vi "SPM Pump v0.7.vi"(0 "Termination char\n(0xA = '\\n' = LF)\n(0xD = '\\r' = CR)":u8=13 format="%.0x", 1 "Enable Termination\nChar (T)":bool=TRUE, 2 "Timeout (ms)":u32=10000, 3 "Serial Settings:Serial End Mode for Reads":u16(ring)=2 items=["None", "LastBit", "TermChar"], 4 "byte count":u32=64, 5 "Delay before read (ms)":u32=1000, 6 "Time <input>":dbl, 7 "error in (no error)":errorcluster, 8 "Serial port input":string="/1ZR", 9 "VISA resource name":refnum<visa-resource-name>="COM6", 10 "parity":u16(ring) items=["None", "Odd", "Even", "Mark", "Space"], 11 "baud rate":u32=9600, 12 "stop bits":u16(ring)=10 items=["1.0"=10, "1.5"=15, "2.0"=20], 13 "data bits":u16=8 min=5 max=8 step=1, 14 "flow control":u16(ring) items=["None"=0, "XON/XOFF"=1, "RTS/CTS"=2, "DTR/DSR"=4], 15 "Time units <input>":string, 19 "Hard stop pump":bool, 20 "Halt pump":bool) -> (16 "Input command":string, 17 "Serial port data":string[](array[string]), 18 "Pump status":string, 23 "Valve position":i32, 24 "Absolute plunger position":i32, 25 "Actual plunger position":i32, 26 "Serial port":string, 27 "error out":errorcluster)   [LabVIEW 2019]
doc: "The Basic Serial Read and Write example performs a Serial Port Read, a Serial Port Write, or a combination of these actions. The user selects the actions (read or write) on the front panel. If both are selected, the VI will write the data first, read data, and then close the VISA session that is opened to the port. This VI will wait until the specified number of bytes is received at the port. Only the number of bytes specified will be read.\n\nINSTRUCTIONS:\n1) Select the serial resource and configuration parameters (baud rate, data bits, parity, stop bits, flow control).\n2) Select the operations to be performed. \n3) Connect the serial port to your device. If no device is available, perform a loopback test by doing one of the following. Short pins 2 and 3 on a RS-232 cable or short pin 4 to pin 8 and pin 5 to pin 9 on a RS-485/422 cable. \n4) Run the VI to see the data read. (The \"read string\" will match the \"string to write\" if a loopback test was performed.)\n\nNote: The parameters set for the serial port must match the parameters of the connected instrument or device. In this example, the bytes to read parameter specifies the number of bytes that the serial port reads. If there were more bytes at the port than the number specified in bytes to read, those bytes would not be read. Also, if you specify to read more bytes than the number of bytes actually read, you might receive a timeout error message.\n\nOn the block diagram, the Configure Serial Port VI sets the configuration parameters. The front panel displays the controls used to configure the basic parameters, such as baud rate, data bits, and parity. Constants configure the other parameters the user probably does not need set. After the VISA Configure Serial Port VI opens the VISA session and configures the port, the VI passes the VISA resource name to other VIs that perform operations on that VISA resource. The VISA Write function sends a command to the serial device and the VISA Read function returns data based on the command. The VISA Close function then closes the reference to the serial device. It is important to close the reference; otherwise communication through with that port through protocols other than VISA might not be possible."
panel:
  in  "Hard stop pump":bool
  in  "Halt pump":bool
  out "Cutoff speed":i32
  out "Maximal speed":i32
  out "Start speed":i32
  # "Select the serial resource and the operations (Read, Write, or both) to be performed.  If both are selected, the VI will write the data first, read data and then close the VISA session that is opened to the port.  This VI will wait until the specified number of bytes is received at the port. Only the number of bytes specified will be read."
  # "For additional information select File >> VI Properties >> Documentation"
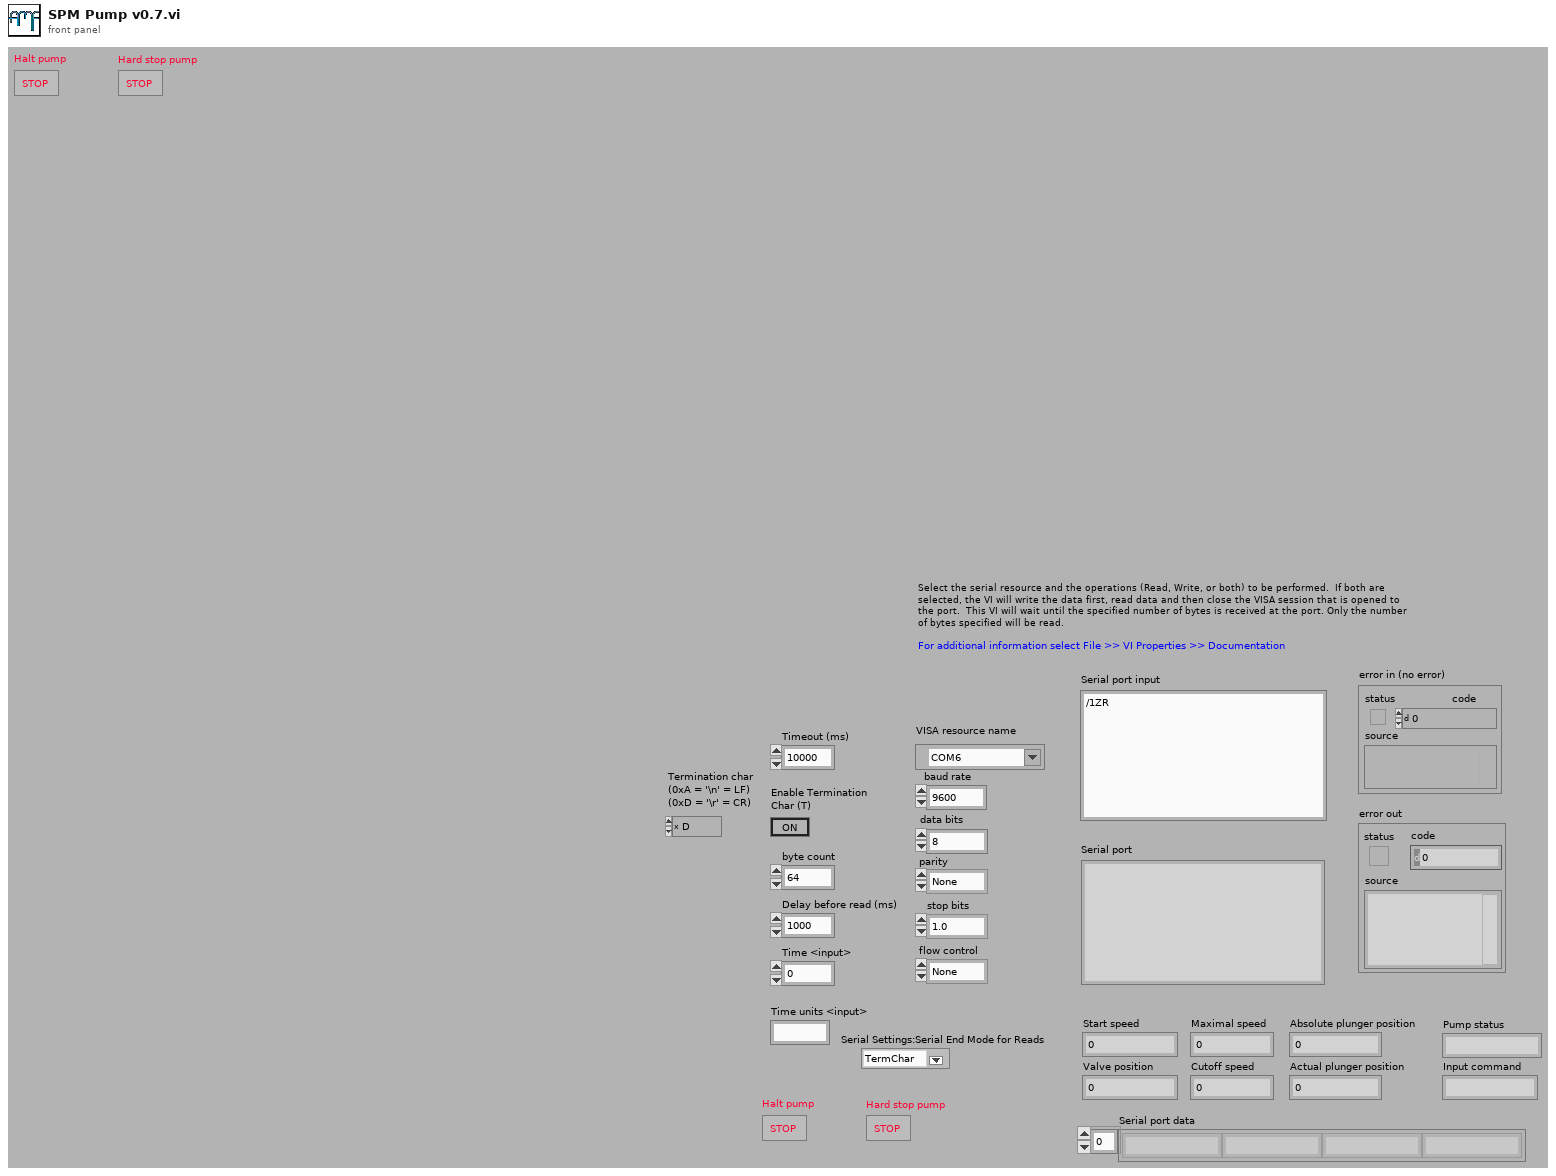
[diagram p1: front panel]
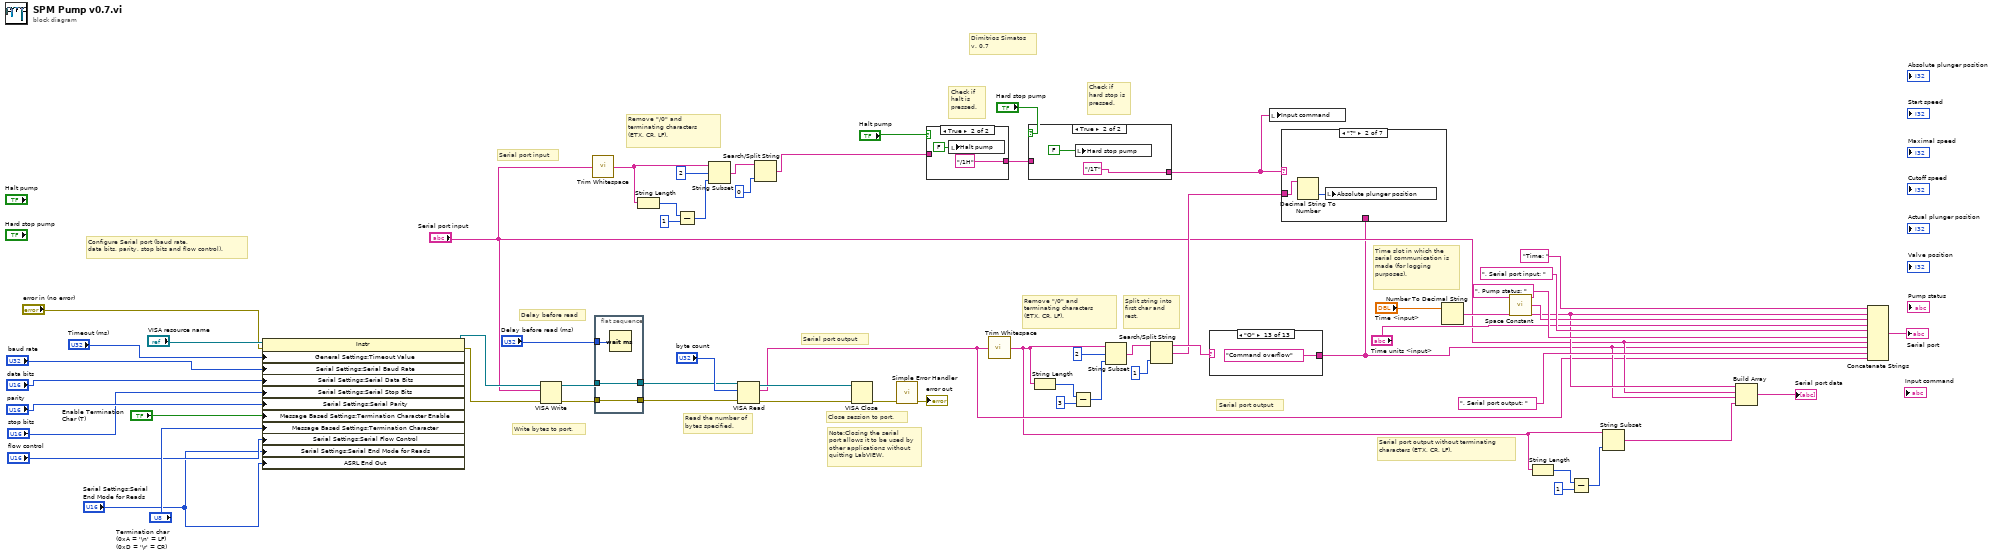
[diagram p0: block diagram]
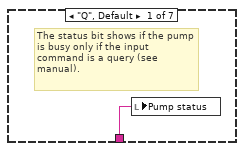
[diagram p4: hidden frame]
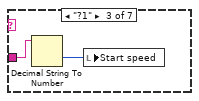
[diagram p5: hidden frame]
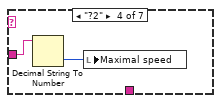
[diagram p6: hidden frame]
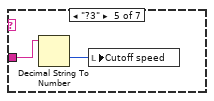
[diagram p7: hidden frame]
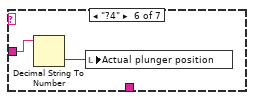
[diagram p8: hidden frame]
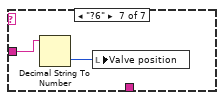
[diagram p9: hidden frame]
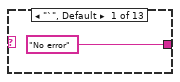
[diagram p10: hidden frame]
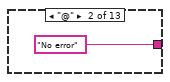
[diagram p11: hidden frame]
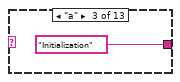
[diagram p12: hidden frame]
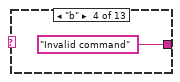
[diagram p13: hidden frame]
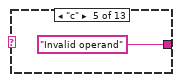
[diagram p14: hidden frame]
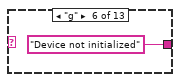
[diagram p15: hidden frame]
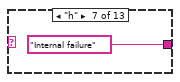
[diagram p16: hidden frame]
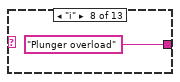
[diagram p17: hidden frame]
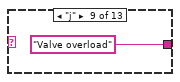
[diagram p18: hidden frame]
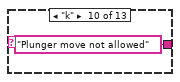
[diagram p19: hidden frame]
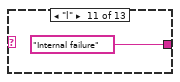
[diagram p20: hidden frame]
diagram:
  # "Check if hard stop is pressed."
  # "Check if halt is pressed."
  # "Serial port output without terminating characters (ETX, CR, LF)."
  # "Serial port input"
  # "Remove \"/0\" and terminating characters (ETX, CR, LF)."
  # "Serial port output"
  # "Serial port output"
  # "Time slot in which the serial communication is made (for logging purposes)."
  # "Split string into first char and rest."
  # "Remove \"/0\" and terminating characters (ETX, CR, LF)."
  # "Delay before read"
  # "Dimitrios Simatos\nv. 0.7"
  # "Read the number of bytes specified."
  # "Write bytes to port."
  # "Note:Closing the serial port allows it to be used by other applications without\nquitting LabVIEW."
  # "Configure Serial port (baud rate,\ndata bits, parity, stop bits and flow control)."
  # "Close session to port."
  n1 = property class="Instr"(reference="VISA resource name", error in="error in (no error)", "General Settings:Timeout Value"="Timeout (ms)", "Serial Settings:Serial Baud Rate"="baud rate", "Serial Settings:Serial Data Bits"="data bits", "Serial Settings:Serial Stop Bits"="stop bits", "Serial Settings:Serial Parity"="parity", "Message Based Settings:Termination Character Enable"="Enable Termination\nChar (T)", "Message Based Settings:Termination Character"="Termination char\n(0xA = '\\n' = LF)\n(0xD = '\\r' = CR)", "Serial Settings:Serial Flow Control"="flow control", "Serial Settings:Serial End Mode for Reads"="Serial Settings:Serial End Mode for Reads", "ASRL End Out"="Serial Settings:Serial End Mode for Reads") -> (reference out=w48:refnum<visa-resource-name>, error out=w47:errorcluster)
  n2 = VISA Write(VISA resource name=w48, write buffer="Serial port input", error in (no error)=w47) -> (VISA resource name out=w43:refnum<visa-resource-name>, error out=w42:errorcluster)  [unwired: 1 out]
  n3 = call <vilib>:"Trim Whitespace.vi"("string"="Serial port input") -> ("trimmed string"=w24:string)  [unwired: 1 in]
  n4 = flat-sequence {
    tunnel: w42 -> [w63]
    tunnel: [w63] -> w41
    tunnel: w43 -> [w62]
    tunnel: [w62] -> w40
    tunnel: "Delay before read (ms)" -> [w64]
    frame #0 {
      n5 = Wait (ms)(milliseconds to wait=w64) -> ()  [unwired: 1 out]
    }
  }
  n6 = String Length(string=w24) -> (length=w28:i32)
  n7 = Subtract(x=w28, y=1) -> (x-y=w27:i32)
  n8 = String Subset(string=w24, offset (0)=2, length (rest)=w27) -> (substring=w22:string)
  n9 = VISA Read(VISA resource name=w40, byte count="byte count", error in (no error)=w41) -> (VISA resource name out=w60:refnum<visa-resource-name>, read buffer=w12:string, error out=w61:errorcluster)  [unwired: 1 out]
  n10 = Search/Split String(string=w22, offset (0)=0) -> (match + rest of string=w1:string)  [unwired: 1 in, 2 out]
  n11 = VISA Close(VISA resource name=w60, error in (no error)=w61) -> (error out=w59:errorcluster)
  n12 = call <vilib>:"Simple Error Handler.vi"("error in (no error)"=w59) -> ("error out"=→"error out":errorcluster)  [unwired: 4 in, 4 out]
  n13 = case shown="True" "Halt pump" {
    tunnel: [w65 "/1H"] -> w5
    tunnel: w1 -> [w65 _]
    frame False {
    }
    frame True {
      n14 = local write "Halt pump"(FALSE) -> ()
    }
  }
  n15 = call <vilib>:"Trim Whitespace.vi"("string"=w12) -> ("trimmed string"=w7:string)  [unwired: 1 in]
  n16 = case shown="True" "Hard stop pump" {
    tunnel: [w68 "/1T"] -> w2
    tunnel: w5 -> [w68 _]
    frame False {
    }
    frame True {
      n17 = local write "Hard stop pump"(FALSE) -> ()
    }
  }
  n18 = String Length(string=w7) -> (length=w38:i32)
  n19 = Subtract(x=w38, y=3) -> (x-y=w37:i32)
  n20 = String Subset(string=w7, offset (0)=2, length (rest)=w37) -> (substring=w11:string)
  n21 = Search/Split String(string=w11, offset (0)=1) -> (substring before match=w33:string, match + rest of string=w21:string)  [unwired: 1 in, 1 out]
  n22 = case shown="\"O\"" w33 {
    tunnel: ["No error" "No error" "Initialization" "Invalid command" "Invalid operand" "Device not initialized" "Internal failure" "Plunger overload" "Valve overload" "Plunger move not allowed" "Internal failure" "A/D converter failure" "Command overflow"] -> w14
    frame "`", Default {
    }
    frame "@" {
    }
    frame "a" {
    }
    frame "b" {
    }
    frame "c" {
    }
    frame "g" {
    }
    frame "h" {
    }
    frame "i" {
    }
    frame "j" {
    }
    frame "k" {
    }
    frame "l" {
    }
    frame "n" {
    }
    frame "O" {
    }
  }
  n23 = local write "Input command"(w2) -> ()
  n24 = case shown="\"?\"" w2 {
    tunnel: w21 -> [_ w85 w87 w90 w91 w94 w96]
    tunnel: w14 -> [w84 _ _ _ _ _ _]
    frame "Q", Default {
      # "The status bit shows if the pump is busy only if the input command is a query (see manual)."
      n25 = local write "Pump status"(w84) -> ()
    }
    frame "?" {
      n26 = Decimal String To Number(string=w85) -> (number=w86:i32)  [unwired: 2 in, 1 out]
      n27 = local write "Absolute plunger position"(w86) -> ()
    }
    frame "?1" {
      n28 = Decimal String To Number(string=w87) -> (number=w88:i32)  [unwired: 2 in, 1 out]
      n29 = local write "Start speed"(w88) -> ()
    }
    frame "?2" {
      n30 = Decimal String To Number(string=w90) -> (number=w89:i32)  [unwired: 2 in, 1 out]
      n31 = local write "Maximal speed"(w89) -> ()
    }
    frame "?3" {
      n32 = Decimal String To Number(string=w91) -> (number=w92:i32)  [unwired: 2 in, 1 out]
      n33 = local write "Cutoff speed"(w92) -> ()
    }
    frame "?4" {
      n34 = Decimal String To Number(string=w94) -> (number=w93:i32)  [unwired: 2 in, 1 out]
      n35 = local write "Actual plunger position"(w93) -> ()
    }
    frame "?6" {
      n36 = Decimal String To Number(string=w96) -> (number=w95:i32)  [unwired: 2 in, 1 out]
      n37 = local write "Valve position"(w95) -> ()
    }
  }
  n38 = Number To Decimal String(number="Time <input>") -> (decimal integer string=w16:string)  [unwired: 1 in]
  n39 = call <vilib>:"Space Constant.vi"() -> ("String"=w17:string)
  n40 = String Length(string=w7) -> (length=w10:i32)
  n41 = Subtract(x=w10, y=1) -> (x-y=w9:i32)
  n42 = String Subset(string=w7, length (rest)=w9) -> (substring=w8:string)  [unwired: 1 in]
  n43 = Build Array(w16, "Serial port input", w14, w8) -> (→"Serial port data":string[])
  n44 = Concatenate Strings("Time: ", w16, w17, "Time units <input>", ", Serial port input: ", "Serial port input", ", Pump status: ", w14, ", Serial port output: ", w12) -> (→"Serial port":string)
